vi "get_context.vi"(8 "error in (no error)":errorcluster, 11 "Log Service in":refnum<class "Log Service.lvclass">) -> (0 "error out":errorcluster, 1 "context":string, 3 "Log Service out":refnum<class "Log Service.lvclass">)   [LabVIEW 2019, in "Utility API.lvlib" / "Log Service.lvclass"]
uses:
  Log Service.lvclass
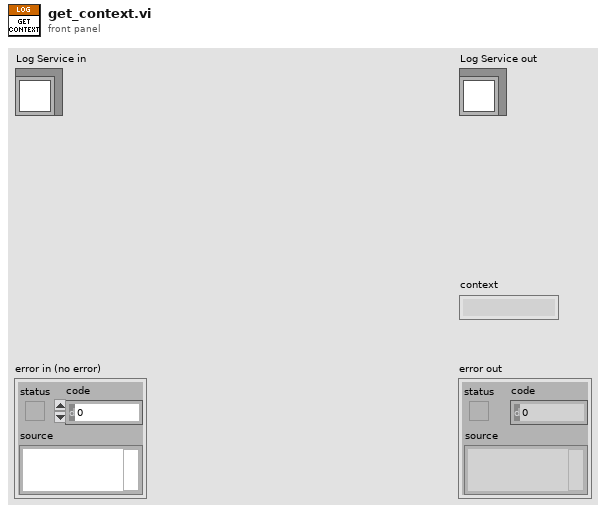
[diagram p1: front panel]
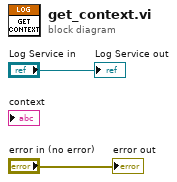
[diagram p0: block diagram]
diagram:
  "error out" <- "error in (no error)"
  "Log Service out" <- "Log Service in"
